vi "PROCESSING PATH (SubVI).vi"(6 "Boolean 3":bool, 9 "Boolean 4":bool, 10 "Boolean 5":bool, 11 "Boolean 6":bool) -> (1 "Boolean":bool, 2 "index of element":i32, 3 "Boolean 2":bool)   [LabVIEW 2021]
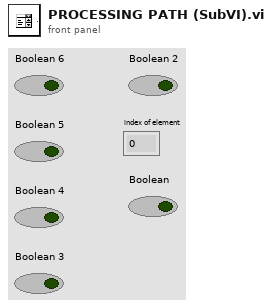
[diagram p1: front panel]
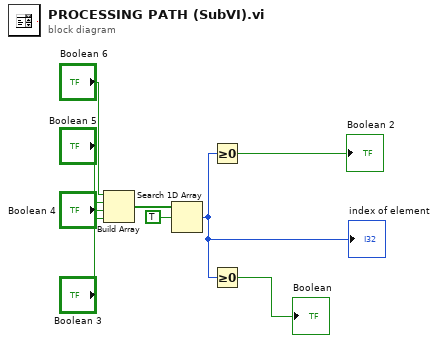
[diagram p0: block diagram]
diagram:
  n1 = Build Array("Boolean 6", "Boolean 5", "Boolean 4", "Boolean 3") -> (w5:bool[])
  n2 = Search 1D Array(1D array=w5, element=TRUE) -> (index of element=w8:i32)  [unwired: 1 in]
  "index of element" <- w8
  n3 = Greater Or Equal To 0?(x=w8) -> (x >= 0?=→"Boolean 2":bool)
  n4 = Greater Or Equal To 0?(x=w8) -> (x >= 0?=→"Boolean":bool)
